vi "RSZVB Acquire Receiver Power Calibration.vi"(4 "Reference Power (0: A Wave)":i32(ring) items=["A Wave", "Nominal"], 5 "Port Number (1)":i32=1, 6 "Source Number (1)":i32=1, 7 "Source (0: Port)":i32(ring) items=["Port"=0, "Generator"=1, "Converter"=12], 8 "error in (no error)":errorcluster {"code" format="%.0x"}, 9 "Wave (0: A)":i32(ring) items=["A", "B", "B1", "B2", "B3", "B4", "B5", "B6", "B7", "B8"], 10 "Channel (1)":i32=1, 11 "VISA session":refnum<visa-resource-name>) -> (0 "error out":errorcluster {"code" format="%.0x"}, 3 "dup VISA session":refnum<visa-resource-name>)   [LabVIEW 2011]
doc: "This function selects the wave quantity and the source for the receiver power calibration, starts the calibration sweep, and applies the receiver power correction.\n\nNote(s):\n\n(1) For some measurements the default set timeout can be insufficient. To set higher timeout use function rszvb_setTimeOut.\n\nRemote-control command(s):\n[SENSe<Ch>:]CORRection:POWer<port_no>:ACQuire AWAVe | BWAVe | B1 | B2 | B3 | B4 | B5 | B6 | B7 | B8[,<cal_port>, PORT | GENerator | CONVerter, <source_no>,AWAVe | NOMinal]"
uses:
  _utility/RSZVB Global Data.vi
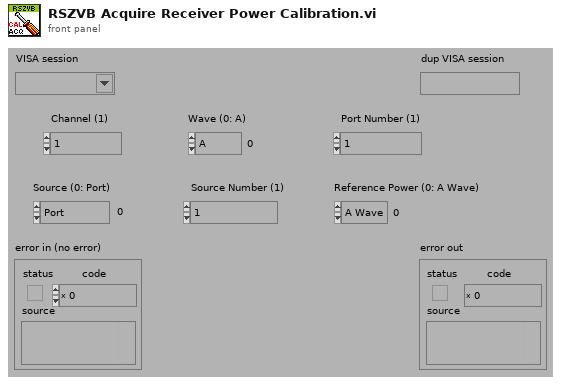
[diagram p1: front panel]
types:
  T1 = cluster{"Error Checking (T: On)":bool, "Installed Options":string[], "Data Valid?":bool, "Ports":i32, "Model":string[], "Option Checking (T: On)":bool}[]
  T2 = cluster{"Error Checking (T: On)":bool, "Installed Options":string[], "Data Valid?":bool, "Ports":i32, "Model":string[], "Option Checking (T: On)":bool}
  T3 = cluster{"Status":bool, "Code":i32, "Source (VI Name)":string}
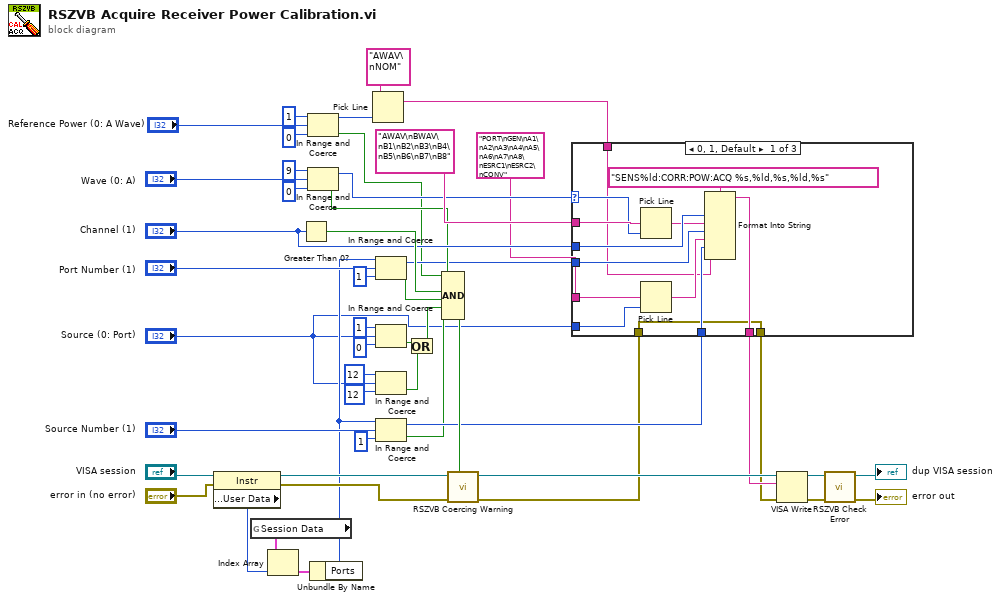
[diagram p0: block diagram]
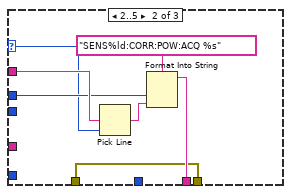
[diagram p2: hidden frame]
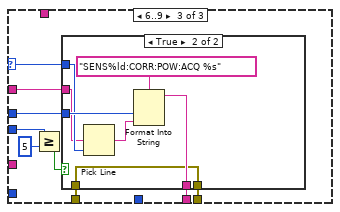
[diagram p3: hidden frame]
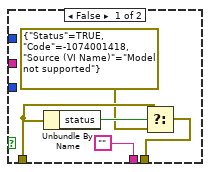
[diagram p4: hidden frame]
diagram:
  n1 = property class="Instr"(reference="VISA session", error in="error in (no error)") -> (reference out=w36:refnum<visa-resource-name>, error out=w37:errorcluster, "General Settings:User Data"=w38:u32)
  n2 = global read "RSZVB Global Data.vi" "Session Data"() -> (w39:T1)
  n3 = Index Array(array=w39, index=w38) -> (element=w40:T2)
  n4 = Greater Than 0?(x="Channel (1)") -> (x > 0?=w44:bool)
  n5 = In Range and Coerce(upper limit=1, x="Reference Power (0: A Wave)", lower limit=0) -> (coerced(x)=w8:i32, In Range?=w9:bool)
  n6 = In Range and Coerce(upper limit=9, x="Wave (0: A)", lower limit=0) -> (coerced(x)=w24:i32, In Range?=w18:bool)
  n7 = Unbundle By Name(w40) -> ("Ports"=w20:i32)
  n8 = Pick Line(multi-line string="AWAV\nNOM", line index=w8) -> (output string=w6:string)  [unwired: 1 in]
  n9 = In Range and Coerce(upper limit=w20, x="Port Number (1)", lower limit=1) -> (coerced(x)=w13:i32, In Range?=w34:bool)
  n10 = In Range and Coerce(upper limit=1, x="Source (0: Port)", lower limit=0) -> (In Range?=w17:bool)  [unwired: 1 out]
  n11 = In Range and Coerce(upper limit=12, x="Source (0: Port)", lower limit=12) -> (In Range?=w3:bool)  [unwired: 1 out]
  n12 = In Range and Coerce(upper limit=w20, x="Source Number (1)", lower limit=1) -> (coerced(x)=w19:i32, In Range?=w16:bool)
  n13 = Or(x=w17, y=w3) -> (x .or. y?=w2:bool)
  n14 = Compound Arithmetic op=AND(w9, w18, w44, w34, w2, w16) -> (w43:bool)
  n15 = call "RSZVB Coercing Warning.vi"("In Range?"=w43, "error in (no error)"=w37, "VISA session"=w36) -> ("error out"=w15:errorcluster, "dup VISA session"=w47:refnum<visa-resource-name>)  [unwired: 7 in]
  n16 = case shown="0, 1, Default" w24 {
    selector: w24 -> [w56 w65 w77]
    tunnel: [w61 w64 w76] -> w42
    tunnel: "Channel (1)" -> [w60 w66 w78]
    tunnel: "AWAV\nBWAV\nB1\nB2\nB3\nB4\nB5\nB6\nB7\nB8" -> [w58 w67 w75]
    tunnel: w13 -> [w59 _ w74]
    tunnel: "PORT\nGEN\nA1\nA2\nA3\nA4\nA5\nA6\nA7\nA8\nESRC1\nESRC2\nCONV" -> [w55 _ _]
    tunnel: "Source (0: Port)" -> [w54 _ _]
    tunnel: w19 -> [w52 _ _]
    tunnel: w15 -> [w51 w63 w71]
    tunnel: [w51 w63 w70] -> w14
    tunnel: w6 -> [w50 _ _]
    frame 0, 1, Default {
      n17 = Pick Line(multi-line string=w58, line index=w56) -> (output string=w57:string)  [unwired: 1 in]
      n18 = Pick Line(multi-line string=w55, line index=w54) -> (output string=w53:string)  [unwired: 1 in]
      n19 = Format Into String(format string="SENS%ld:CORR:POW:ACQ %s,%ld,%s,%ld,%s", w60, w57, w59, w53, w52, w50) -> (resulting string=w61:string)  [unwired: 2 in, 1 out]
    }
    frame 2..5 {
      n20 = Pick Line(multi-line string=w67, line index=w65) -> (output string=w68:string)  [unwired: 1 in]
      n21 = Format Into String(format string="SENS%ld:CORR:POW:ACQ %s", w66, w68) -> (resulting string=w64:string)  [unwired: 2 in, 1 out]
    }
    frame 6..9 {
      n22 = Greater Or Equal?(x=w74, y=5) -> (x >= y?=w72:bool)
      n23 = case shown="True" w72 {
        tunnel: w78 -> [_ w88]
        tunnel: w77 -> [_ w87]
        tunnel: ["" w86] -> w76
        tunnel: w75 -> [_ w85]
        tunnel: w71 -> [w82 w84]
        tunnel: [w80 w84] -> w70
        frame False {
          n24 = Unbundle By Name(w82) -> ("status"=w83:bool)
          n25 = Select(t=w82, s=w83, f=T3 {"Status"=TRUE, "Code"=-1074001418, "Source (VI Name)"="Model not supported"}) -> (s? t:f=w80:T3)
        }
        frame True {
          n26 = Pick Line(multi-line string=w85, line index=w87) -> (output string=w89:string)  [unwired: 1 in]
          n27 = Format Into String(format string="SENS%ld:CORR:POW:ACQ %s", w88, w89) -> (resulting string=w86:string)  [unwired: 2 in, 1 out]
        }
      }
    }
  }
  n28 = VISA Write(VISA resource name=w47, write buffer=w42, error in (no error)=w14) -> (VISA resource name out=w45:refnum<visa-resource-name>, error out=w46:errorcluster)  [unwired: 1 out]
  n29 = call "RSZVB Check Error.vi"("error in (no error)"=w46, "VISA session"=w45) -> ("error out"=→"error out":errorcluster, "dup VISA session"=→"dup VISA session":refnum<visa-resource-name>)  [unwired: 8 in]
